vi "FUG_PowerSupply.SetVoltage.vi"(0 "i ref in":refnum<vi>, 2 "value":dbl, 5 "error in (no error)":errorcluster, 7 "channelIndex":i32) -> (14 "i ref out":refnum<vi>, 19 "error out (no error)":errorcluster)   [LabVIEW 2014, in "FUG_PowerSupply.lvlib"]
doc: "This VI calculates the right current from the DB values, saves the actual set current to the I-Attribute and set´s the Set Current-Service."
uses:
  FUG_PowerSupply.lvlib
  CSCore/CSSystem/CoreDefs/CoreDefs.error_type.ctl
  CSCore/CSSystem/CoreDefs/CoreDefs.error_severity.ctl
  CSCore/CSApplicationBaseClasses/PSChannelBase/PSChannelBase.directionType.ctl
  CSCore/CSApplicationBaseClasses/PSChannelBase/PSChannelBase.serviceType.ctl
  CSlibraries/UtilityLib/UtilityLib.valueStatus.ctl
  CSCore/CSSystem/CoreLib/CoreLib.lvlib
  CSlibraries/UtilityLib/UtilityLib.lvlib
  CSCore/CSApplicationBaseClasses/PSChannelBase/PSChannelBase.lvlib
  CSlibraries-extern/DimLVEvent/LVDimInterface/LVDimInterface.lvlib
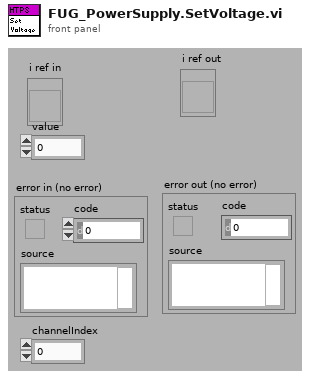
[diagram p1: front panel]
types:
  T1 = typedef "CoreDefs.error_severity.ctl" = enum16{"undefined", "information", "warning", "error", "fatal"}
  T2 = typedef "CoreDefs.error_type.ctl" = enum16{"no error", "can't load process", "can't unload process", "process does not exist", "can't install process", "can't remove process", "unknown function", "time out", "can't execute function", "duplicate queue name", "super not found", "caller queue invalid", "can't ping process", "unknown error", "VISA Error", "VISA timeout", "GPIB timeout", "GPIB error", "communication error", "data type mismatch", "can't read data from OPC server", "can't write data to OPC server", "OET error", "function not implemented", "process already exists", "invalid Shared Variable name", "error writing Shared Variable", "error reading Shared Variable", "invalid client name", "corrupt database", "unknown class", "call not authorized", "parameter out of range", "OET timeout: can't get data to modify", "invalid queue name", "requested operation incompatible with current state", "event undefined", "event disabled", "state undefined", "caller is not a friend", "EventBuilder: bad eventID", "EventBuilder: no DAQ devices", "a thread must not stop itself", "UNUSED ELEMENT4", "DiscArchiver: eventData incomplete", "DiscArchiver: eventData does not belong to run", "DiscArchiver: can't open file", "DiscArchiver: can't write to file", "DiscArchiver: available disc space low", "can't acquire semaphore", "error reading data from database", "notifier object is not existing", "can't register process", "can't unregister process", "illegal event type", "object disabled", "object already exists", "can't change state", "Instrument not found", "no connection to remote node", "invalid reference", "N/A", "UNUSED ELEMENT 1", "element not found", "illegal TCP/IP connection detected", "object does not exist", "invalid access ID", "unknown CS system", "invalid privilige", "unsupported data type", "unsupported server type", "IO server already exists", "Shared Variable already exists"}
  T3 = typedef "UtilityLib.lvlib/UtilityLib.valueStatus.ctl" = enum16{"no info available", "stand by/off", "on", "warning", "alarm/malfunction", "not implemented", "user action required", "important information", "system default", "control default", "indicator default", "button default"}
  T4 = typedef "PSChannelBase.lvlib/PSChannelBase.serviceType.ctl" = enum16{"onOff", "voltage", "current", "tripCurrent", "rampUpSpeed", "rampDownSpeed", "status"}
  T5 = typedef "PSChannelBase.lvlib/PSChannelBase.directionType.ctl" = enum16{"unknown", "update actual value", "update nominal value", "update both"}
  T6 = typedef "FUG_PowerSupply.lvlib/FUG_PowerSupply.i attribute.ctl" = cluster{"Type":string, "Elektrode Name":string, "CALC_FACTOR_SET_VOLTAGE":dbl, "CALC_FACTOR_GET_VOLTAGE":dbl, "CALC_FACTOR_GET_CURRENT":dbl, "CALC_FACTOR_SET_CURRENT ":dbl, "REG_VALUE":dbl, "Sign":bool, "setVoltID":i32, "setCurrentID":i32, "setPowerOnID":i32, "MaxVoltage":dbl}
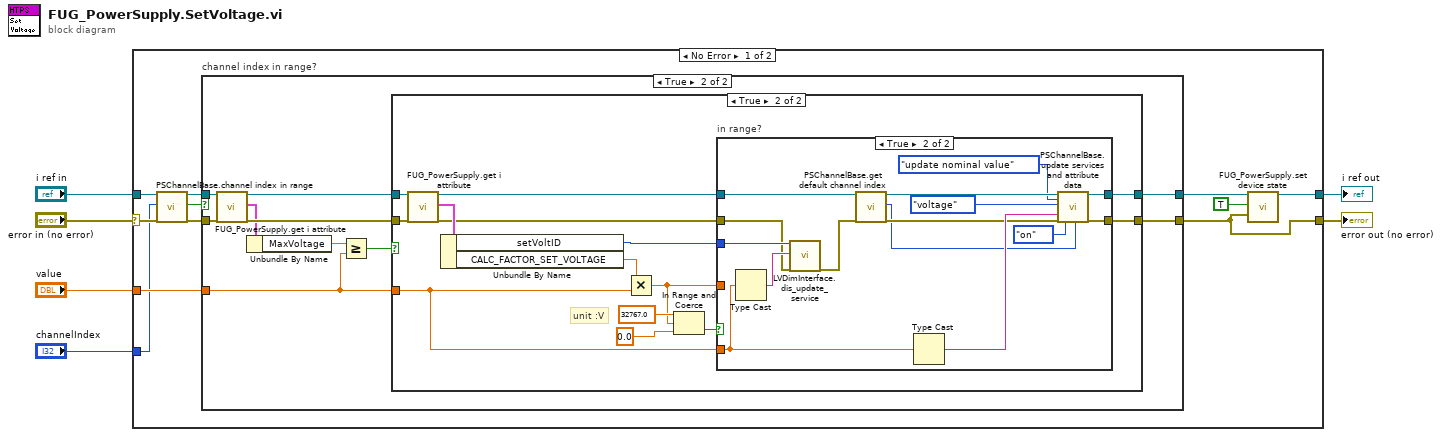
[diagram p0: block diagram]
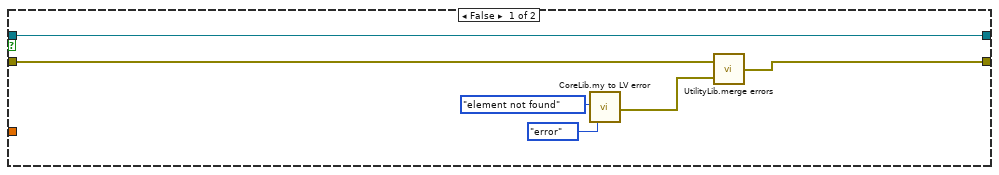
[diagram p2: hidden frame]
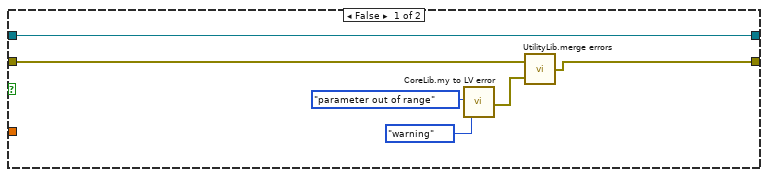
[diagram p3: hidden frame]
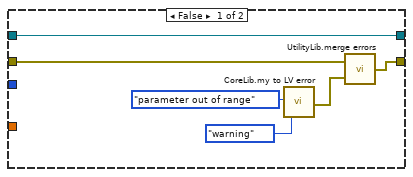
[diagram p4: hidden frame]
diagram:
  n1 = case shown="No Error" "error in (no error)" {
    selector: "error in (no error)" -> [w16 w76]
    tunnel: [w9 w76] -> w3
    tunnel: "i ref in" -> [w15 w75]
    tunnel: [w8 w75] -> w5
    tunnel: "value" -> [w17 _]
    tunnel: "channelIndex" -> [w14 _]
    frame No Error {
      n2 = call "PSChannelBase.channel index in range.vi"("i ref in"=w15, "channelIndex"=w14, "error in (no error)"=w16) -> ("i ref out"=w11:refnum<vi>, "in range"=w12:bool, "error out"=w13:errorcluster)  [unwired: 14 in]
      n3 = case "channel index in range?" shown="True" w12 {
        tunnel: w11 -> [w23 w29]
        tunnel: [w23 w33] -> w10
        tunnel: w13 -> [w20 w31]
        tunnel: [w18 w32] -> w9
        tunnel: w17 -> [_ w24]
        frame False {
          n4 = call "CoreLib.my to LV error.vi"("ErrorTypes"=CoreDefs.error_type."element not found", "severityLevel"=CoreDefs.error_severity."error") -> ("myErrorCluster"=w19:errorcluster)  [unwired: 16 in, 1 out]
          n5 = call "UtilityLib.merge errors.vi"("error2 (no error)"=w19, "error1 (no error)"=w20) -> ("error out"=w18:errorcluster)
        }
        frame True {
          n6 = call "FUG_PowerSupply.get i attribute.vi"("i ref in"=w29, "error in (no error)"=w31) -> ("i ref out"=w28:refnum<vi>, "i attribute"=w27:T6, "error out"=w30:errorcluster)  [unwired: 15 in]
          n7 = Unbundle By Name(w27) -> ("MaxVoltage"=w25:dbl)
          n8 = Greater Or Equal?(x=w25, y=w24) -> (x >= y?=w26:bool)
          n9 = case shown="True" w26 {
            tunnel: w28 -> [w34 w47]
            tunnel: [w34 w46] -> w33
            tunnel: w30 -> [w36 w45]
            tunnel: [w35 w44] -> w32
            tunnel: w24 -> [_ w40]
            frame False {
              n10 = call "CoreLib.my to LV error.vi"("ErrorTypes"=CoreDefs.error_type."parameter out of range", "severityLevel"=CoreDefs.error_severity."warning") -> ("myErrorCluster"=w37:errorcluster)  [unwired: 16 in, 1 out]
              n11 = call "UtilityLib.merge errors.vi"("error2 (no error)"=w37, "error1 (no error)"=w36) -> ("error out"=w35:errorcluster)
            }
            frame True {
              # "unit :V"
              n12 = call "FUG_PowerSupply.get i attribute.vi"("i ref in"=w47, "error in (no error)"=w45) -> ("i ref out"=w42:refnum<vi>, "i attribute"=w53:T6, "error out"=w43:errorcluster)  [unwired: 15 in]
              n13 = Unbundle By Name(w53) -> ("setVoltID"=w41:i32, "CALC_FACTOR_SET_VOLTAGE"=w52:dbl)
              n14 = Multiply(x=w52, y=w40) -> (x*y=w48:dbl)
              n15 = In Range and Coerce(upper limit=32767.0, x=w48, lower limit=0.0 ("upper limit")) -> (In Range?=w51:bool)  [unwired: 1 out]
              n16 = case "in range?" shown="True" w51 {
                tunnel: w43 -> [w57 w62]
                tunnel: [w55 w73] -> w44
                tunnel: w48 -> [_ _]
                tunnel: w42 -> [w54 w71]
                tunnel: [w54 w74] -> w46
                tunnel: w41 -> [_ w64]
                tunnel: w40 -> [_ w60]
                frame False {
                  n17 = call "CoreLib.my to LV error.vi"("ErrorTypes"=CoreDefs.error_type."parameter out of range", "severityLevel"=CoreDefs.error_severity."warning") -> ("myErrorCluster"=w56:errorcluster)  [unwired: 16 in, 1 out]
                  n18 = call "UtilityLib.merge errors.vi"("error2 (no error)"=w56, "error1 (no error)"=w57) -> ("error out"=w55:errorcluster)
                }
                frame True {
                  n19 = Type Cast(x=w60) -> (*(type *) &x=w63:string)  [unwired: 1 in]
                  n20 = call "LVDimInterface.dis_update_service.vi"("my_serviceID"=w64, "data"=w63, "error in (no error)"=w62) -> ("error out"=w61:errorcluster)  [unwired: 14 in, 2 out]
                  n21 = call "PSChannelBase.get default channel index.vi"("i ref in"=w71, "error in (no error)"=w61) -> ("i ref out"=w70:refnum<vi>, "defaultChannelIndex"=w68:i32, "error out"=w69:errorcluster)  [unwired: 15 in]
                  n22 = Type Cast(x=w60) -> (*(type *) &x=w72:string)  [unwired: 1 in]
                  n23 = call "PSChannelBase.update services and attribute data.vi"("i ref in"=w70, "direction"=PSChannelBase.directionType."update nominal value", "service"=PSChannelBase.serviceType."voltage", "value"=w72, "error in (no error)"=w69, "quality"=UtilityLib.valueStatus."on", "channelNumber"=w68) -> ("i ref out"=w74:refnum<vi>, "error out"=w73:errorcluster)  [unwired: 10 in, 1 out]
                }
              }
            }
          }
        }
      }
      n24 = call "FUG_PowerSupply.set device state.vi"("i ref in"=w10, "implicit"=TRUE, "device error"=w9) -> ("i ref out"=w8:refnum<vi>)  [unwired: 14 in, 2 out]
    }
    frame Error {
    }
  }
  "error out (no error)" <- w3
  "i ref out" <- w5
